vi "Single_Wire_Gate.vi"(6 "2x2 Unitary Matrix":cdb[][](array[numeric]), 8 "error in (no error)":errorcluster, 9 "d CtrlLine in":refnum<class "CtrlLine.lvclass">, 10 "u CtrlLine in":refnum<class "CtrlLine.lvclass">, 11 "QuWire in":refnum<class "QuWire.lvclass">) -> (0 "error out":errorcluster, 3 "QuWire out":refnum<class "QuWire.lvclass">)   [LabVIEW 2020, in "QuWire.lvclass"]
uses:
  QuWire.lvclass
  CtrlLine/CtrlLine.lvclass
  QuWire.lvclass/QuWire.ctl
  SimAlg/PrllPerElement/PrllPerElmnt.lvclass
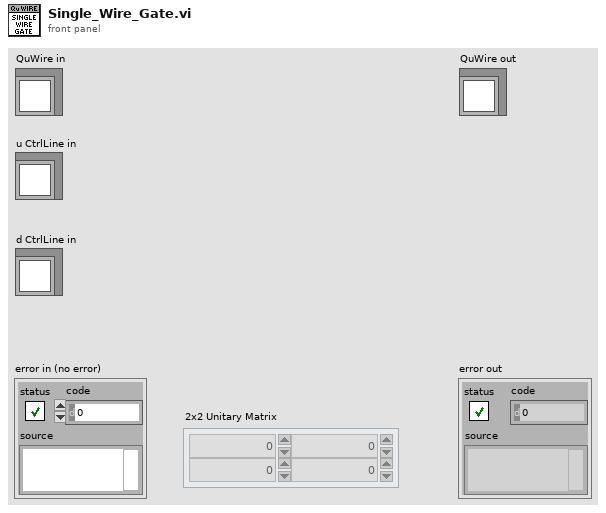
[diagram p1: front panel]
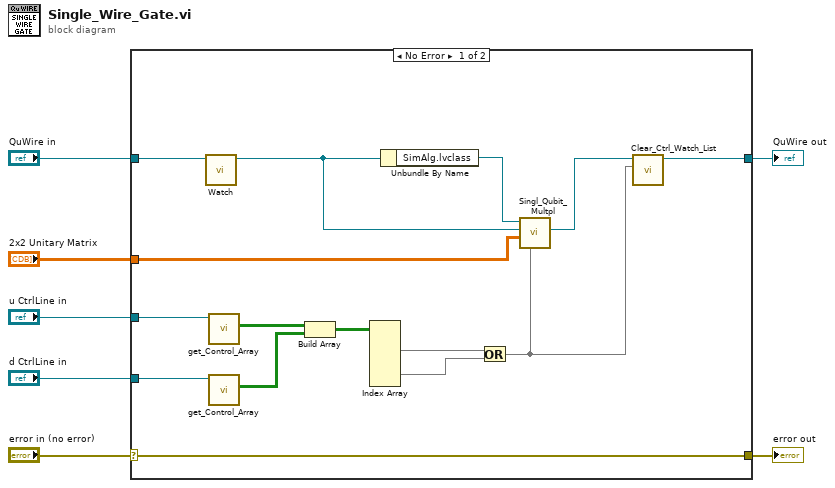
[diagram p0: block diagram]
diagram:
  n1 = case shown="No Error" "error in (no error)" {
    selector: "error in (no error)" -> [w22 w24]
    tunnel: [w22 w24] -> w6
    tunnel: [w17 w23] -> w4
    tunnel: "QuWire in" -> [w18 w23]
    tunnel: "2x2 Unitary Matrix" -> [w21 _]
    tunnel: "u CtrlLine in" -> [w20 _]
    tunnel: "d CtrlLine in" -> [w19 _]
    frame No Error {
      n2 = call "Watch.vi"("QuWire in"=w18) -> ("QuWire out"=w10:refnum<class "QuWire.lvclass">)  [unwired: 9 in, 1 out]
      n3 = call "get_Control_Array.vi"("CtrlLine in"=w20) -> ("Control Array"=w16:bool[][])  [unwired: 8 in, 2 out]
      n4 = call "get_Control_Array.vi"("CtrlLine in"=w19) -> ("Control Array"=w15:bool[][])  [unwired: 8 in, 2 out]
      n5 = Build Array(w16, w15) -> (w14:bool[][][])
      n6 = Index Array(array=w14) -> (element #1=w13:bool[][], element #2=w12:bool[][])  [unwired: 6 in]
      n7 = Unbundle By Name(w10) -> ("SimAlg.lvclass"=w11:refnum<class "PrllPerElmnt.lvclass">)
      n8 = Or(x=w13, y=w12) -> (x .or. y?=w8:bool[][])
      n9 = call-dynamic "Singl_Qubit_Multpl.vi"("Control Bitmask"=w8, "2x2 Unitary Matrix"=w21, "QuWire in"=w10, "SimAlg in"=w11) -> ("QuWire out"=w9:refnum<class "QuWire.lvclass">)  [unwired: 5 in, 2 out]
      n10 = call "Clear_Ctrl_Watch_List.vi"("Control Array"=w8, "QuWire in"=w9) -> ("QuWire out"=w17:refnum<class "QuWire.lvclass">)  [unwired: 9 in]
    }
    frame Error {
    }
  }
  "error out" <- w6
  "QuWire out" <- w4
